vi "Actor Core.vi"(8 "error in":errorcluster, 11 "DAQ in":refnum<class "DAQ.lvclass">) -> (0 "error out":errorcluster, 3 "Actor out":refnum<class "Actor.lvclass">)   [LabVIEW 2020, in "DAQ.lvlib" / "DAQ.lvclass"]
doc: "(<B>Filename</B>: Actor Framework.lvlib:Actor.lvclass:Actor Core.vi)\n\nReceives messages to the actor, reacts to them, and initiates any error handling that may shut the actor down.\n\nDescendant classes may override this VI to append parallel tasks for the actor to complete while it handles messages. Overrides use the Call Parent Class Method node."
uses:
  DAQ.lvclass
  C:/Program Files/National Instruments/LabVIEW 2020/vi.lib/ActorFramework/Actor/Actor.lvclass
  <vilib>/ActorFramework/Actor/Actor.lvclass
  DAQ Controller/DAQ Controller.lvclass
  DAQ.lvclass/DAQ.ctl
  Device/Device/Device.lvclass
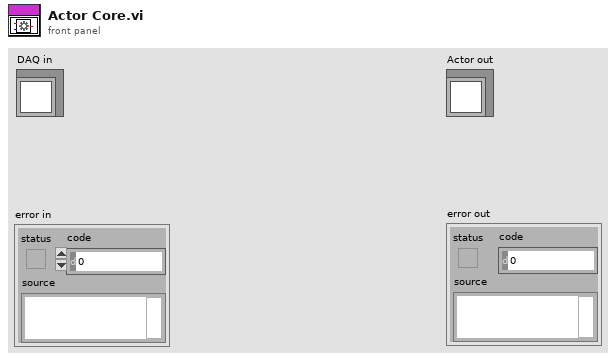
[diagram p1: front panel]
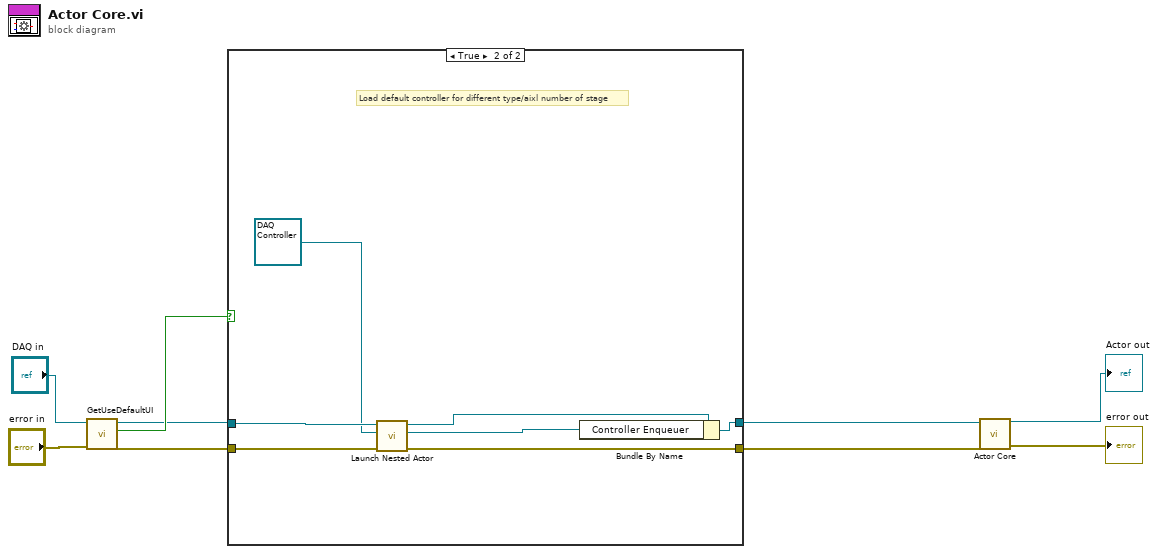
[diagram p0: block diagram]
diagram:
  n1 = call-dynamic "GetUseDefaultUI.vi"("error in (no error)"="error in", "Device in"="DAQ in") -> ("error out"=w3:errorcluster, "User Default UI?"=w5:bool, "Device out"=w4:refnum<class "DAQ.lvclass">)  [unwired: 7 in]
  n2 = case shown="True" w5 {
    tunnel: [w11 w16] -> w1
    tunnel: [w10 w17] -> w2
    tunnel: w4 -> [w11 w15]
    tunnel: w3 -> [w10 w14]
    frame False {
    }
    frame True {
      # "Load default controller for different type/aixl number of stage"
      n3 = call <vilib>:"Launch Nested Actor.vi"("error in (no error)"=w14, "Nested Actor"=refnum<class "DAQ Controller.lvclass"> refnum ("DAQ.lvlib:DAQ Controller.lvlib:DAQ Controller.lvclass"), "Caller Actor in"=w15) -> ("error out"=w17:errorcluster, "Nested Actor's Enqueuer"=w18:refnum<class "Message Enqueuer.lvclass">, "Caller Actor out"=w13:refnum<class "DAQ.lvclass">)  [unwired: 6 in]
      n4 = Bundle By Name(cluster=w13, "Controller Enqueuer"=w18) -> (w16:refnum<class "DAQ.lvclass">)
    }
  }
  n5 = call-parent "Actor Core.vi"("error in"=w2, "Actor in"=w1) -> ("error out"=→"error out":errorcluster, "Actor out"=→"Actor out":refnum<class "Actor.lvclass">)  [unwired: 8 in]
